vi "Create File Response.vi"(8 "error in (no error)":errorcluster, 11 "Path":path) -> (0 "error out":errorcluster, 3 "File Response out":refnum<class "File Response.lvclass">)   [LabVIEW 2020, in "HTTP Server.lvlib" / "File Response.lvclass"]
uses:
  File Response.lvclass
  File Response.lvclass/File Response.ctl
  <vilib>/IlluminatedG/IG HTTP Utils/HTTP Utils/Response/Response.lvclass
  C:/Program Files (x86)/National Instruments/LabVIEW 2020/vi.lib/IlluminatedG/IG HTTP Utils/HTTP Utils/Response/Response.lvclass
  C:/dev/IlluminatedG/lv-http-server/HTTP Server/File Response/File Response.lvclass
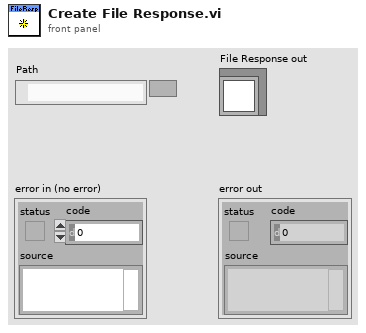
[diagram p1: front panel]
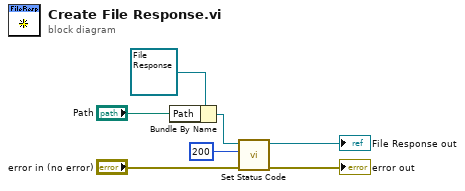
[diagram p0: block diagram]
diagram:
  n1 = Bundle By Name(cluster=refnum<class "File Response.lvclass"> refnum ("File Response in"), "Path"="Path") -> (w5:refnum<class "File Response.lvclass">)
  n2 = call <vilib>:"Set Status Code.vi"("error in (no error)"="error in (no error)", "Status Code"=u16 200, "Response in"=w5) -> ("error out"=→"error out":errorcluster, "Response out"=→"File Response out":refnum<class "File Response.lvclass">)  [unwired: 7 in]
